vi "Process Monkey Report.vi"(8 "error in (no error)":errorcluster, 10 "Monkey Status Message":T1, 11 "Tamer in":refnum<class "Tamer.lvclass">=refnum) -> (0 "error out":errorcluster, 3 "Tamer out":refnum<class "Tamer.lvclass">)   [LabVIEW 2020, in "CIRCUS_uServices.lvlib" / "Holy Trinity.lvlib" / "Tamer.lvlib" / "Tamer.lvclass"]
uses:
  Tamer.lvclass
  Link Chain GUI.ctl
  Monkey Summary.ctl
  TALOS/TALOS_PPL.lvlibp/Father of all uServices/Father of all uServices/Father of all uServices.lvclass
  TALOS/TALOS_PPL.lvlibp
  Run Utilities/TypeDefs/Monkey Status.ctl
  Run Utilities/Run Utilities.lvlib
  TALOS/TALOS_PPL.lvlibp/Father of all uServices/Father of all uServices/Children Methods/Get GUI Item Value - Variant.vi
  C:/Users/marco/Documents/GitHub_Lab/CIRCUS/TALOS/TALOS_PPL.lvlibp/Ancestor/Ancestor/Ancestor.lvclass
  C:/Users/marco/Documents/GitHub_Lab/CIRCUS/TALOS/Actor Framework.lvlibp/1abvi3w/vi.lib/ActorFramework/Actor/Actor.lvclass
  C:/Users/marco/Documents/GitHub_Lab/CIRCUS/TALOS/TALOS_PPL.lvlibp/Father of all uServices/Father of all uServices/Father of all uServices.lvclass
  Run Utilities/Schedule/Schedule.lvclass
  Run Utilities/TypeDefs/Messages/Monkey Status Message.ctl
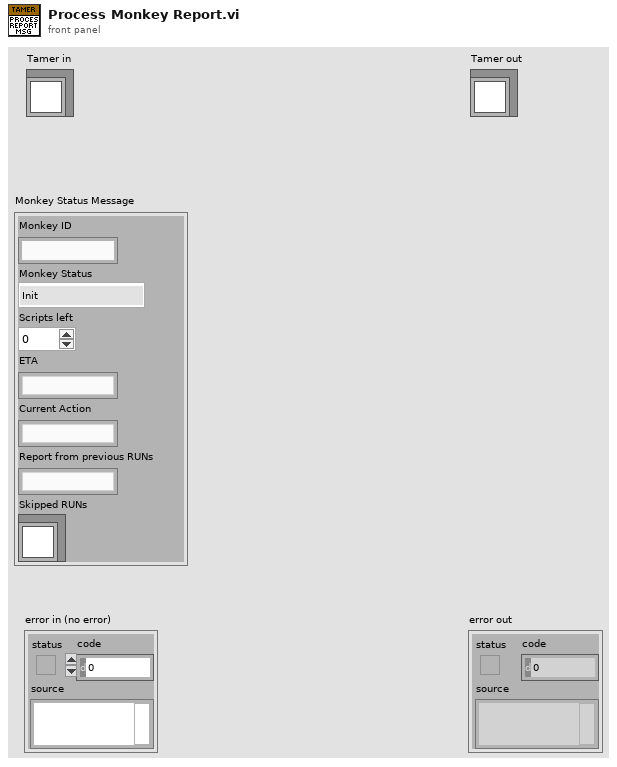
[diagram p1: front panel]
types:
  T1 = typedef "CIRCUS_uServices.lvlib/Run Utilities.lvlib/Monkey Status Message.ctl" = cluster{"Monkey ID":string, "Monkey Status":T2, "Scripts left":u32, "ETA":string, "Current Action":string, "Report from previous RUNs":string, "Skipped RUNs":refnum<class "Schedule.lvclass">}
  T2 = typedef "CIRCUS_uServices.lvlib/Run Utilities.lvlib/Monkey Status.ctl" = enum16{"Init", "Paused", "Ongoing", "Stopped", "Finished (no errors)", "Finished (with errors)"}
  T3 = typedef "CIRCUS_uServices.lvlib/Holy Trinity.lvlib/Tamer.lvlib/Tamer.lvclass/Monkey Summary.ctl" = cluster{"Color":u32, "Status":T2, "Continuous":bool, "Scripts left":u32, "Scripts skipped":u32, "ETA":string, "Current Action":string, "Report from previous RUNs":string, "Monkey ID":string, "With DAQ?":bool, "Linked?":T4, "Paused":bool}
  T4 = typedef "CIRCUS_uServices.lvlib/Holy Trinity.lvlib/Tamer.lvlib/Tamer.lvclass/Link Chain GUI.ctl" = bool
  T5 = typedef "TALOS.lvlib/Run Utilities.lvlib/Monkey Status.ctl" = enum16{"Init", "Paused", "Ongoing", "Stopped", "Finished (no errors)", "Finished (with errors)"}
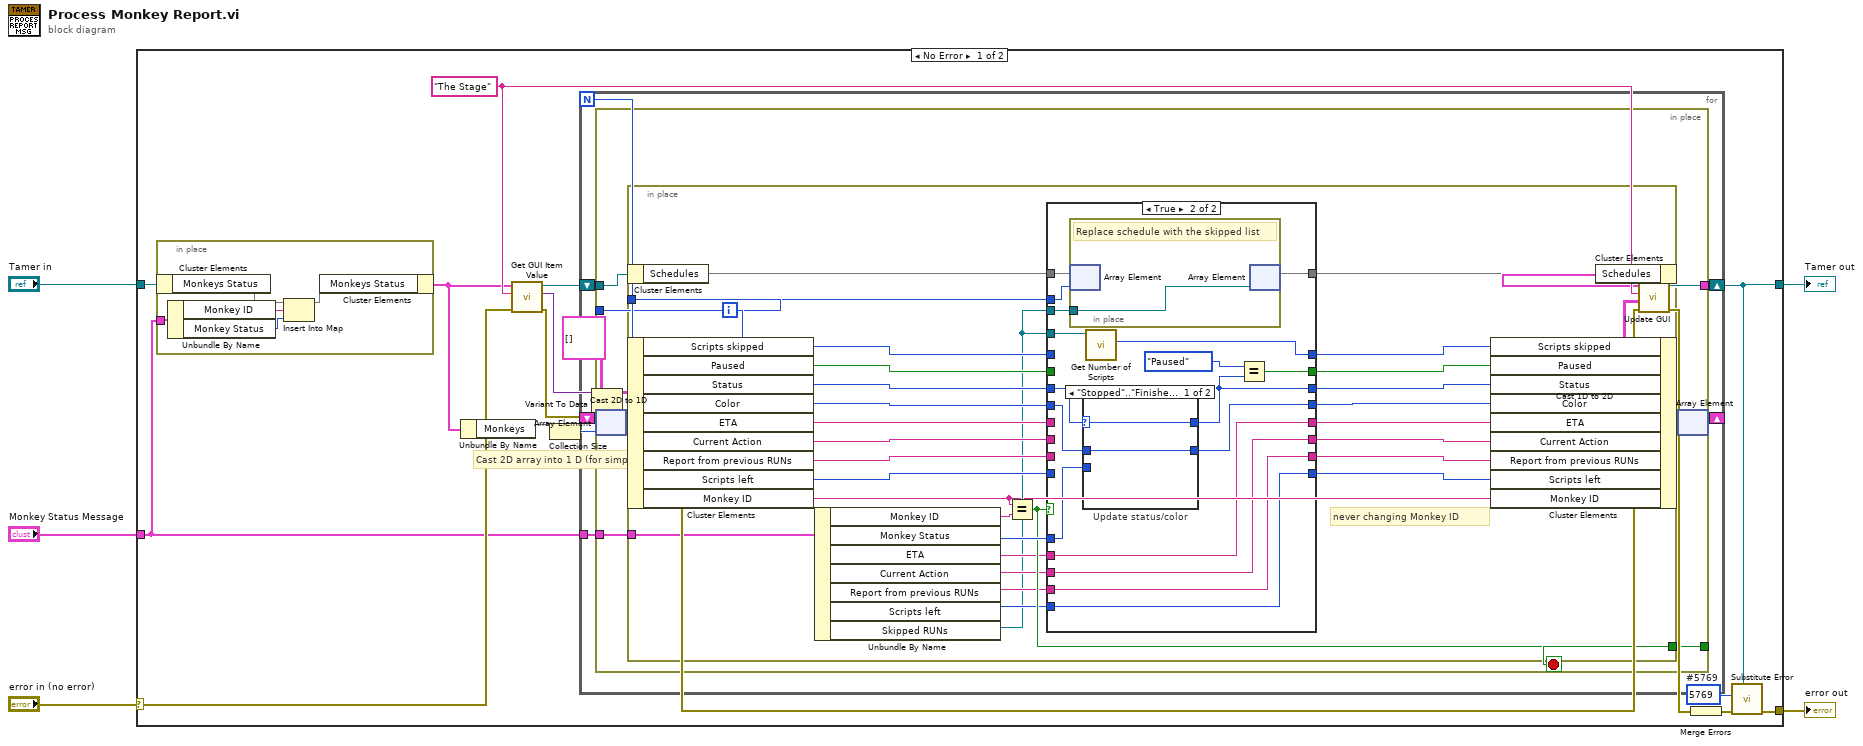
[diagram p0: block diagram]
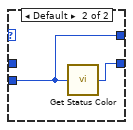
[diagram p3: hidden frame]
diagram:
  n1 = case shown="No Error" "error in (no error)" {
    selector: "error in (no error)" -> [w23 w108]
    tunnel: [w27 w108] -> w4
    tunnel: [w9 w107] -> w2
    tunnel: "Tamer in" -> [w8 w107]
    tunnel: "Monkey Status Message" -> [w6 _]
    frame No Error {
      w13 = "The Stage" ("FP Item Name")
      w26 = 5769  # #5769
      # "Re-cast 1D array into 2D"
      # "Cast 2D array into 1 D (for simplicity)"
      n2 = in-place {
        in-place-border: w6 -> [w30]
        n3 = in-place-cluster #1(w8) -> ("Monkeys Status"=w32)
        n4 = Unbundle By Name(w30) -> ("Monkey ID"=w29:string, "Monkey Status"=w28:T2)
        n5 = Insert Into Map(map in=w32, key=w29, value=w28) -> (map out=w31:map{string, T5})  [unwired: 2 out]
        n6 = in-place-cluster #1("Monkeys Status"=w31) -> (w7:cluster{})
      }
      n7 = Unbundle By Name(w7) -> ("Monkeys"=w16)
      n8 = call-poly "Get GUI Item Value.vi"("error in (no error)"=w23, "FP Item Name"=w13, "uService Template in"=w7) -> ("error out"=w17:errorcluster, "Value"=w19:variant, "uService Template out"=w12:refnum<class "Father of all uServices.lvclass">)  [unwired: 6 in]
      n9 = Collection Size(1:w16) -> (0:w11:i32)
      n10 = Variant To Data(error in=w17, type=T3[][] [] ("2D Synchronous Monkeys"), Variant=w19) -> (data=w18:T3[][], error out=w21:errorcluster)
      n11 = call "Cast 2D to 1D.vi"("1D size"=w11, "2D Synchronous Monkeys"=w18) -> ("1D Synchronous Monkeys"=w22:T3[])
      n12 = for {
        N: w11 -> [_]
        tunnel: w6 -> [w39]
        shift-right: [w36] -> w10
        shift-left: w12 -> [w37]
        shift-right: [w33] -> w20
        shift-left: w22 -> [w35]
        i -> [w34]
        stop <- w38 stop-if-true
        n13 = in-place {
          in-place-border: w39 -> [w46]
          in-place-border: [w45] -> w38
          in-place-border: w37 -> [w44]
          in-place-border: w34 -> [w43]
          in-place-border: [w42] -> w36
          n14 = in-place-array #2(w35, w34) -> (w41:T3)
          n15 = in-place {
            in-place-border: w46 -> [w72]
            in-place-border: [w71] -> w45
            in-place-border: w43 -> [w52]
            # "never changing Monkey ID"
            n16 = in-place-cluster #3(w44) -> ("Schedules"=w54)
            n17 = in-place-cluster #4(w41) -> ("Scripts skipped"=w73:u32, "Paused"=w51:bool, "Status"=w70:T2, "Color"=w67:u32, "ETA"=w66:string, "Current Action"=w64:string, "Report from previous RUNs"=w62:string, "Scripts left"=w60:u32, "Monkey ID"=w49:string)
            n18 = Unbundle By Name(w72) -> ("Monkey ID"=w74:string, "Monkey Status"=w75:T2, "ETA"=w58:string, "Current Action"=w57:string, "Report from previous RUNs"=w56:string, "Scripts left"=w55:u32, "Skipped RUNs"=w50:refnum<class "Schedule.lvclass">)
            n19 = Equal?(x=w49, y=w74) -> (x = y?=w71:bool)
            n20 = case shown="True" w71 {
              tunnel: [w83 w90] -> w68
              tunnel: w75 -> [_ w91]
              tunnel: w70 -> [w84 w92]
              tunnel: [w84 w87] -> w69
              tunnel: w67 -> [w83 w89]
              tunnel: w66 -> [w82 _]
              tunnel: [w82 w101] -> w65
              tunnel: w64 -> [w81 _]
              tunnel: [w81 w100] -> w63
              tunnel: w62 -> [w80 _]
              tunnel: [w80 w99] -> w61
              tunnel: w60 -> [w79 _]
              tunnel: [w79 w98] -> w59
              tunnel: w58 -> [_ w101]
              tunnel: w57 -> [_ w100]
              tunnel: w56 -> [_ w99]
              tunnel: w55 -> [_ w98]
              tunnel: w54 -> [w78 w97]
              tunnel: [w78 w96] -> w53
              tunnel: w50 -> [_ w95]
              tunnel: w52 -> [_ w93]
              tunnel: w51 -> [w76 _]
              tunnel: w50 -> [_ w94]
              tunnel: w73 -> [w77 _]
              tunnel: [w77 w88] -> w48
              tunnel: [w76 w86] -> w47
              frame False {
              }
              frame True {
                n21 = in-place {
                  in-place-border: w95 -> [w106]
                  # "Replace schedule with the skipped list"
                  n22 = in-place-array #5(w97, w93) -> ()  [unwired: 1 out]
                  n23 = in-place-array #5(w106) -> (w96)  [unwired: 1 out]
                }
                n24 = case "Update status/color" shown="\"Stopped\"..\"Finished (with errors)\"" w92 {
                  selector: w92 -> [w103 _]
                  tunnel: w91 -> [_ w104]
                  tunnel: [w102 w105] -> w90
                  tunnel: [w103 w104] -> w87
                  tunnel: w89 -> [w102 _]
                  frame "Stopped".."Finished (with errors)" {
                  }
                  frame Default {
                    n25 = call "Get Status Color.vi"("Monkey Status"=w104) -> ("Color"=w105:u32)
                  }
                }
                n26 = call-dynamic "Get Number of Scripts.vi"("Schedule in"=w94) -> ("No. of Scripts"=w88:u32)  [unwired: 8 in, 2 out]
                n27 = Equal?(x=Monkey_Status."Paused", y=w87) -> (x = y?=w86:bool)
              }
            }
            n28 = in-place-cluster #4("Scripts skipped"=w48, "Paused"=w47, "Status"=w69, "Color"=w68, "ETA"=w65, "Current Action"=w63, "Report from previous RUNs"=w61, "Scripts left"=w59, "Monkey ID"=w49) -> (w40:T3)
            n29 = in-place-cluster #3("Schedules"=w53) -> (w42:cluster{})
          }
          n30 = in-place-array #2(w40) -> (w33:T3[])  [unwired: 1 out]
        }
      }
      n31 = call "Cast 1D to 2D.vi"("1D Monkeys"=w20) -> ("2D Monkeys"=w14:T3[][])
      n32 = call "Update GUI.vi"("error in (no error)"=w21, "Data"=w14, "GUI Item Name"=w13, "uService Template in"=w10) -> ("error out"=w25:errorcluster, "uService Template out"=w9:refnum<class "Father of all uServices.lvclass">)  [unwired: 6 in]
      n33 = Merge Errors(w25) -> (w24:errorcluster)
      n34 = call "Substitute Error.vi"("LabVIEW Object"=w9, "error in (no error)"=w24, "Error Code"=w26) -> ("error out"=w27:errorcluster)  [unwired: 8 in]
    }
    frame Error {
    }
  }
  "error out" <- w4
  "Tamer out" <- w2
